vi "Stop Calculation.vi"(8 "error in (no error)":errorcluster, 10 "appended array":T1[](array[typedef]) {"Zoom Parameters"."fwidth:" format="%#_6p"; "Zoom Parameters"."f0:" format="%#_6p"}, 11 "GPU FFT Calculator in":refnum<class "GPU FFT Calculator.lvclass">) -> (0 "error out":errorcluster, 3 "GPU FFT Calculator out":refnum<class "GPU FFT Calculator.lvclass">)   [LabVIEW 2020, in "GPU FFT Calculator.lvlib" / "GPU FFT Calculator.lvclass"]
uses:
  GPU FFT Calculator.lvclass
  C:/Program Files/National Instruments/LabVIEW 2026/vi.lib/ActorFramework/Actor/Actor.lvclass
  C:/Users/natan/Documents/G2CPU-Performance-Demo/Calculation Worker/Calculation Worker/Calculation Worker.lvclass
  GPU Calculation Message.ctl
  <vilib>/Natan Biesmans/G2CPU GPU and CPU HPC Toolkit/G2CPU Libraries/Async IO/DMA Manager/DMA Manager.lvclass
  <vilib>/Natan Biesmans/G2CPU GPU and CPU HPC Toolkit/G2CPU Libraries/Arrays/1DArray/s16/1D Array s16.lvclass
  <vilib>/Natan Biesmans/G2CPU GPU and CPU HPC Toolkit/G2CPU Libraries/Arrays/1DArray/f32/1D Array f32.lvclass
  chart zoom.ctl
  GPU Metrics.ctl
  <vilib>/ActorFramework/Actor/Actor.lvclass/Actor.ctl
  Application Manager/Application Manager Messages/Set UI GPU Done Msg/Set UI GPU Done Msg.lvclass/Set UI GPU Done Msg.ctl
  <vilib>/ActorFramework/Message Enqueuer/Message Enqueuer.lvclass/Message Enqueuer.ctl
  GPU FFT Calculator Messages/Start Calculation Msg/Start Calculation Msg.lvclass/Start Calculation Msg.ctl
  <vilib>/ActorFramework/Message Enqueuer/Enqueue.vi
  <vilib>/ActorFramework/Message Enqueuer/Init from Existing Queue.vi
  Application Manager/Application Manager Messages/Set UI GPU Done Msg/Set UI GPU Done Msg.lvclass
  C:/Program Files/National Instruments/LabVIEW 2026/vi.lib/ActorFramework/Message/Message.lvclass
  GPU FFT Calculator Messages/Start Calculation Msg/Start Calculation Msg.lvclass
  <vilib>/ActorFramework/Message Priority Queue/Priority Enqueue.vi
  <vilib>/ActorFramework/Message Enqueuer/Message Enqueuer.lvclass
  <vilib>/ActorFramework/Actor/Actor.lvclass
  Simple UI/Simple UI/Simple UI.lvclass
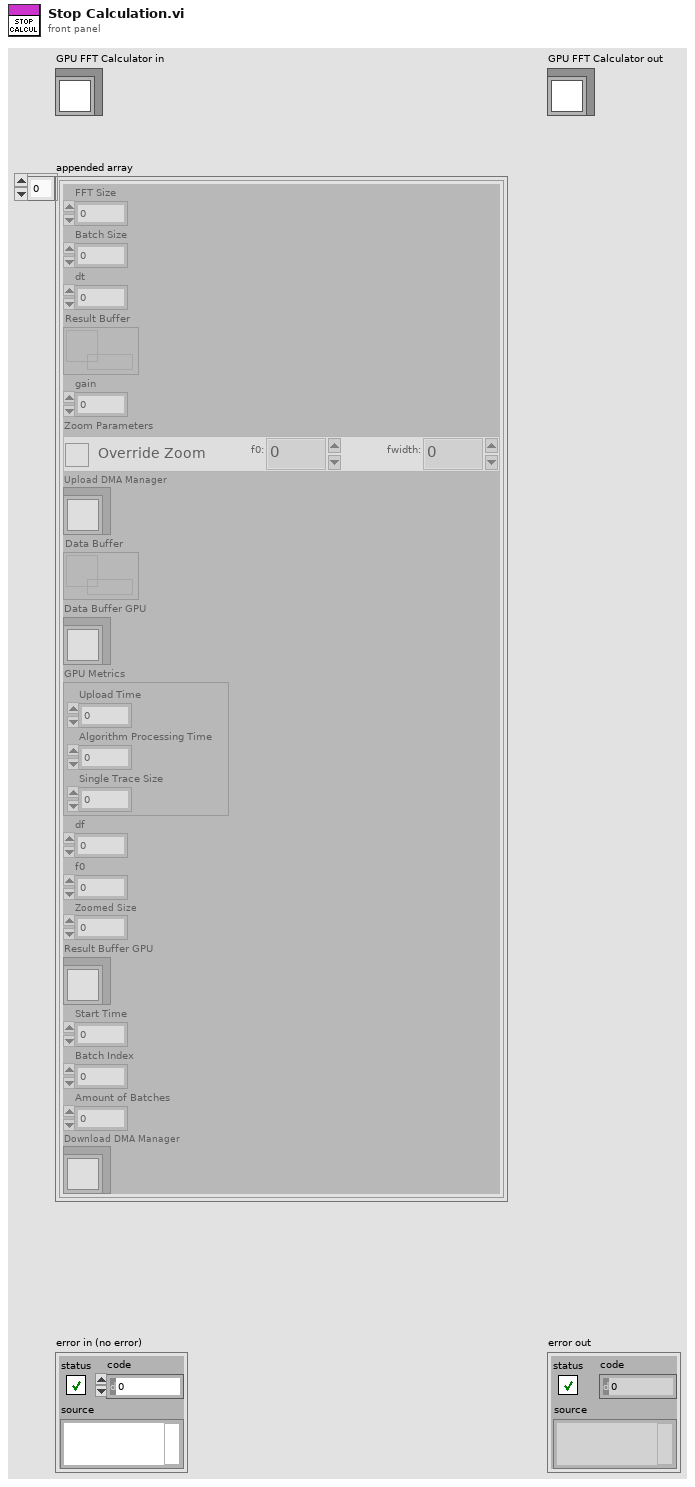
[diagram p1: front panel]
types:
  T1 = typedef "GPU FFT Calculator.lvlib/GPU FFT Calculator.lvclass/GPU Calculation Message.ctl" = cluster{"FFT Size":u64, "Batch Size":u64, "dt":dbl, "Result Buffer":refnum<data-value>, "gain":dbl, "Zoom Parameters":T2, "Upload DMA Manager":refnum<class "DMA Manager.lvclass">, "Data Buffer":refnum<data-value>, "Data Buffer GPU":refnum<class "1D Array s16.lvclass">, "GPU Metrics":T3, "df":dbl, "f0":dbl, "Zoomed Size":u64, "Result Buffer GPU":refnum<class "1D Array f32.lvclass">, "Start Time":dbl, "Batch Index":i32, "Amount of Batches":i32, "Download DMA Manager":refnum<class "DMA Manager.lvclass">}
  T2 = typedef "Simple UI.lvlib/Simple UI.lvclass/chart zoom.ctl" = cluster{"Override":bool, "f0: ":dbl, "fwidth: ":dbl}
  T3 = typedef "GPU FFT Calculator.lvlib/GPU FFT Calculator.lvclass/GPU Metrics.ctl" = cluster{"Upload Time":dbl, "Algorithm Processing Time":dbl, "Single Trace Size":u64}
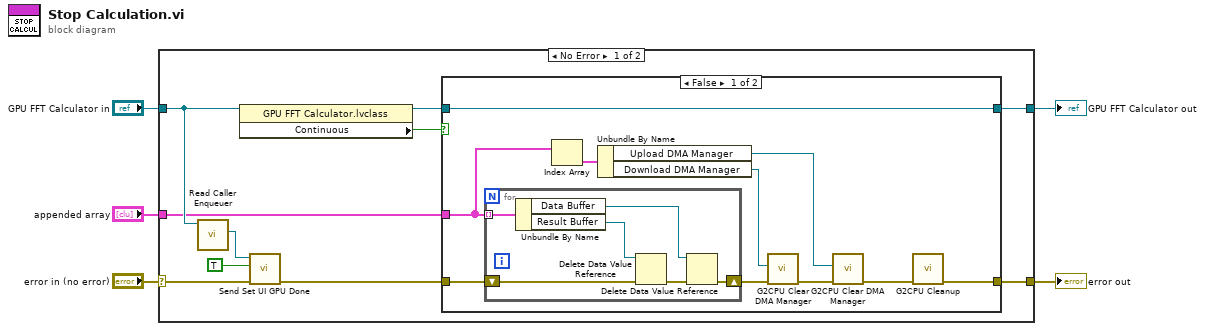
[diagram p0: block diagram]
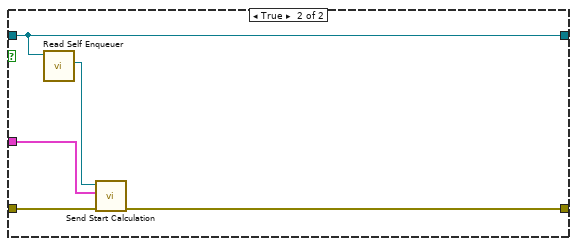
[diagram p2: hidden frame]
diagram:
  n1 = case shown="No Error" "error in (no error)" {
    selector: "error in (no error)" -> [w7 w38]
    tunnel: [w8 w38] -> w4
    tunnel: [w9 w37] -> w2
    tunnel: "GPU FFT Calculator in" -> [w15 w37]
    tunnel: "appended array" -> [w6 _]
    frame No Error {
      n2 = call <vilib>:"Read Caller Enqueuer.vi"("Actor"=w15) -> ("Caller Enqueuer"=w14:refnum<class "Message Enqueuer.lvclass">)  [unwired: 10 in]
      n3 = property class="GPU FFT Calculator.lvclass"(reference=w15) -> (reference out=w10:refnum<class "GPU FFT Calculator.lvclass">, "Continuous"=w11:bool)  [unwired: 1 in, 1 out]
      n4 = call "Send Set UI GPU Done.vi"("error in (no error)"=w7, "GPU Done"=TRUE, "Message Enqueuer"=w14) -> ("error out"=w12:errorcluster)  [unwired: 7 in, 1 out]
      n5 = case shown="False" w11 {
        tunnel: w12 -> [w24 w34]
        tunnel: w10 -> [w25 w36]
        tunnel: [w25 w36] -> w9
        tunnel: [w16 w33] -> w8
        tunnel: w6 -> [w23 w32]
        frame False {
          n6 = for {
            shift-right: [w26] -> w17
            shift-left: w24 -> [w28]
            tunnel: w23 -> [w31] mode=indexing
            n7 = Unbundle By Name(w31) -> ("Data Buffer"=w29:refnum<data-value>, "Result Buffer"=w30:refnum<data-value>)
            n8 = Delete Data Value Reference(data value reference=w30, error in=w28) -> (error out=w27:errorcluster)  [unwired: 1 out]
            n9 = Delete Data Value Reference(data value reference=w29, error in=w27) -> (error out=w26:errorcluster)  [unwired: 1 out]
          }
          n10 = Index Array(array=w23) -> (element=w22:T1)  [unwired: 1 in]
          n11 = Unbundle By Name(w22) -> ("Upload DMA Manager"=w20:refnum<class "DMA Manager.lvclass">, "Download DMA Manager"=w21:refnum<class "DMA Manager.lvclass">)
          n12 = call <vilib>:"G2CPU Clear DMA Manager.vi"("error in (no error)"=w17, "DMA Manager"=w21) -> ("error out"=w19:errorcluster)  [unwired: 9 in]
          n13 = call <vilib>:"G2CPU Clear DMA Manager.vi"("error in (no error)"=w19, "DMA Manager"=w20) -> ("error out"=w18:errorcluster)  [unwired: 9 in]
          n14 = call <vilib>:"G2CPU Cleanup.vi"("error in (no error)"=w18) -> ("error out"=w16:errorcluster)  [unwired: 10 in]
        }
        frame True {
          n15 = call <vilib>:"Read Self Enqueuer.vi"("Actor"=w36) -> ("Self Enqueuer"=w35:refnum<class "Message Enqueuer.lvclass">)  [unwired: 10 in]
          n16 = call "Send Start Calculation.vi"("error in (no error)"=w34, "appended array"=w32, "Message Enqueuer"=w35) -> ("error out"=w33:errorcluster)  [unwired: 7 in, 1 out]
        }
      }
    }
    frame Error {
    }
  }
  "error out" <- w4
  "GPU FFT Calculator out" <- w2
